vi "clLabview_version.vi"(0 "vi_lib.lvlib:clLabview.lvclass":refnum<class "clLabview.lvclass">) -> (11 "version_text":string, 13 "version_info":string, 14 "major":u8=3 min=1 max=99 step=1, 15 "minor":u8 max=99 step=1, 16 "bugfix":u8 step=1, 17 "build":u8 step=1, 18 "stage":u8(ring) items=["development", "alpha", "beta", "release"], 19 "flags":i32 step=1)   [LabVIEW 2011, in "vi_lib.lvlib" / "clLabview.lvclass"]
uses:
  clLabview.lvclass
  clFileReader/clFileReader.lvclass
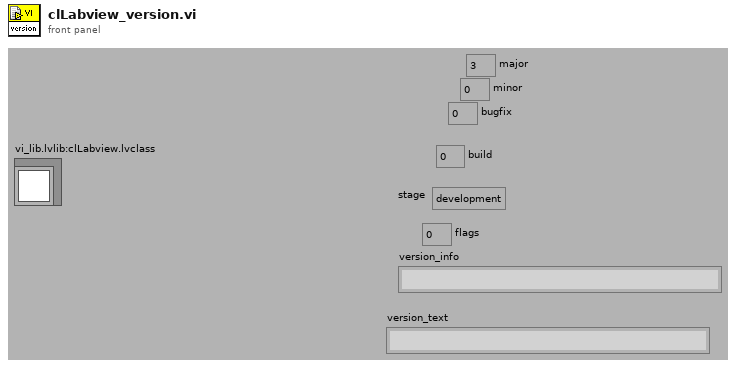
[diagram p1: front panel]
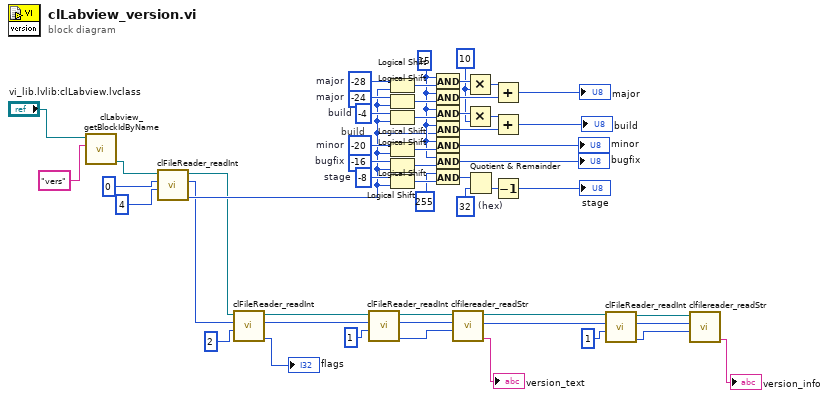
[diagram p0: block diagram]
diagram:
  w31 = 32  # (hex)
  w41 = 15
  w42 = i8 -4  # build
  w43 = i8 -8  # stage
  w44 = i8 -16  # bugfix
  w45 = i8 -20  # minor
  w46 = i8 -24  # major
  w47 = i8 -28  # major
  w32 = 10
  # "build"
  n1 = call "clLabview_getBlockIdByName.vi"("Block Name"="vers", "vi_lib.lvlib:clLabview.lvclass"="vi_lib.lvlib:clLabview.lvclass") -> ("Block Content"=w22:refnum<class "clFileReader.lvclass">)  [unwired: 2 in, 6 out]
  n2 = call "clFileReader_readInt.vi"("size"=u32 4, "offset"=u32 0, "clFileReader.lvclass IN"=w22) -> ("OUT Value"=w19:u32, "new offset"=w18:u32, "clFileReader.lvclass OUT"=w15:refnum<class "clFileReader.lvclass">)  [unwired: 6 out]
  n3 = call "clFileReader_readInt.vi"("size"=u32 2, "offset"=w18, "clFileReader.lvclass IN"=w15) -> ("OUT Value"=→"flags":u32, "new offset"=w13:u32, "clFileReader.lvclass OUT"=w14:refnum<class "clFileReader.lvclass">)  [unwired: 6 out]
  n4 = call "clFileReader_readInt.vi"("size"=u32 1, "offset"=w13, "clFileReader.lvclass IN"=w14) -> ("OUT Value"=w9:u32, "new offset"=w10:u32, "clFileReader.lvclass OUT"=w11:refnum<class "clFileReader.lvclass">)  [unwired: 6 out]
  n5 = Logical Shift(y=w47, x=w19) -> (x << y=w53:u32)
  n6 = Logical Shift(y=w46, x=w19) -> (x << y=w52:u32)
  n7 = Logical Shift(y=w42, x=w19) -> (x << y=w48:u32)
  n8 = Logical Shift(y=w45, x=w19) -> (x << y=w51:u32)
  n9 = Logical Shift(y=w44, x=w19) -> (x << y=w50:u32)
  n10 = Logical Shift(y=w43, x=w19) -> (x << y=w49:u32)
  n11 = And(x=w41, y=w53) -> (x .and. y?=w35:u32)
  n12 = And(x=w41, y=w52) -> (x .and. y?=w38:u32)
  n13 = And(x=w41, y=w48) -> (x .and. y?=w34:u32)
  n14 = And(x=w41, y=w19) -> (x .and. y?=w36:u32)
  n15 = And(x=w41, y=w51) -> (x .and. y?=→"minor":u32)
  n16 = And(x=w41, y=w50) -> (x .and. y?=→"bugfix":u32)
  n17 = And(x=255, y=w49) -> (x .and. y?=w33:u32)
  n18 = call "clfilereader_readStr.vi"("size"=w9, "offset"=w10, "clFileReader.lvclass IN"=w11) -> ("ReadStr - OUT Value"=→"version_text":string, "new offset"=w4:u32, "clFileReader.lvclass OUT"=w7:refnum<class "clFileReader.lvclass">)  [unwired: 6 out]
  n19 = Multiply(x=w35, y=w32) -> (x*y=w39:u32)
  n20 = Multiply(x=w34, y=w32) -> (x*y=w37:u32)
  n21 = Quotient & Remainder(x=w33, y=w31) -> (floor(x/y)=w30:u32)  [unwired: 1 out]
  n22 = Add(x=w39, y=w38) -> (x+y=→"major":u32)
  n23 = Add(x=w37, y=w36) -> (x+y=→"build":u32)
  n24 = Decrement(x=w30) -> (x-1=→"stage":u32)
  n25 = call "clFileReader_readInt.vi"("size"=u32 1, "offset"=w4, "clFileReader.lvclass IN"=w7) -> ("OUT Value"=w2:u32, "new offset"=w5:u32, "clFileReader.lvclass OUT"=w6:refnum<class "clFileReader.lvclass">)  [unwired: 6 out]
  n26 = call "clfilereader_readStr.vi"("size"=w2, "offset"=w5, "clFileReader.lvclass IN"=w6) -> ("ReadStr - OUT Value"=→"version_info":string)  [unwired: 8 out]
